vi "Analog Output (FPGA).vi"() -> ()   [LabVIEW 2012]
doc: "This VI will continually write single point values to 4 channels."
uses:
  <vilib>/rvi/eio/common/nirviEmuTemplateMethod_errors.vi
  <vilib>/eio/EIONode/EIONode.xnode
panel:
  in  "stop":bool
  in  "AO Data":T1
  out "FPGA Error Out":errorcluster
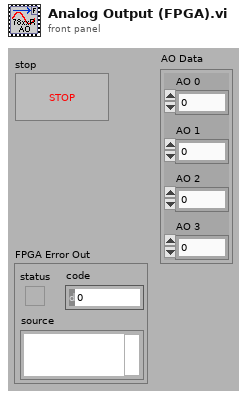
[diagram p1: front panel]
types:
  T1 = cluster{"AO 0":i16, "AO 1":i16, "AO 2":i16, "AO 3":i16}
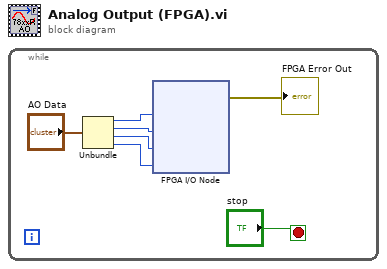
[diagram p0: block diagram]
diagram:
  n1 = while {
    stop <- "stop" stop-if-true
    n2 = Unbundle("AO Data") -> ("AO 0"=w4:i16, "AO 1"=w3:i16, "AO 2"=w2:i16, "AO 3"=w1:i16)
    n3 = xnode "FPGA I/O Node"("AO0"=w4, "AO1"=w3, "AO2"=w2, "AO3"=w1) -> ("error out"=→"FPGA Error Out":errorcluster)  [unwired: 5 in, 4 out]
  }
